vi "Optimiertes Array zusammenstutzen.vi"(6 "Speicher Freigeben":bool, 8 "Zeitstempeln":timestamp[](array[timestamp]), 10 "Anzahl Elemente":i32, 11 "Messdaten":sgl[][](array[numeric])) -> (0 "Zeitstempeln":timestamp[](array[timestamp]), 3 "Messdaten":sgl[][](array[numeric]))   [LabVIEW 2020, in "Messdaten.lvlib"]
uses:
  Messdaten.lvlib
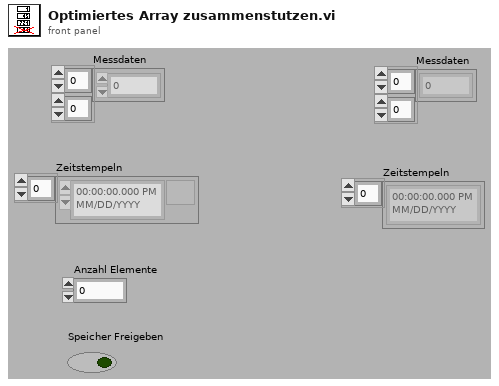
[diagram p1: front panel]
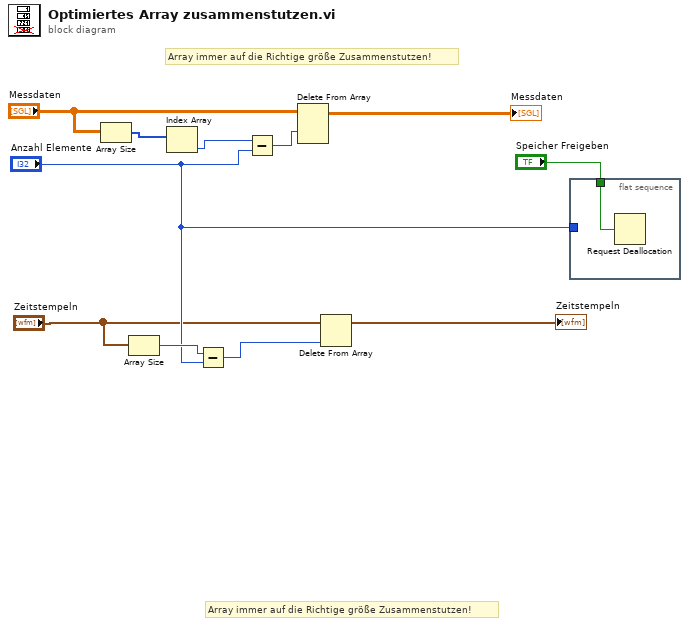
[diagram p0: block diagram]
diagram:
  # "Array immer auf die Richtige größe Zusammenstutzen!"
  # "Array immer auf die Richtige größe Zusammenstutzen!"
  n1 = Array Size(array="Messdaten") -> (size(s)=w8:i32[])
  n2 = Array Size(array="Zeitstempeln") -> (size(s)=w4:i32)
  n3 = Index Array(array=w8) -> (element=w7:i32)  [unwired: 1 in]
  n4 = Subtract(x=w4, y="Anzahl Elemente") -> (x-y=w1:i32)
  n5 = Subtract(x=w7, y="Anzahl Elemente") -> (x-y=w5:i32)
  n6 = Delete From Array(array="Messdaten", index (row)=w5) -> (array with subset deleted=→"Messdaten":sgl[][])  [unwired: 2 in, 1 out]
  n7 = Delete From Array(array="Zeitstempeln", index=w1) -> (array with subset deleted=→"Zeitstempeln":timestamp[])  [unwired: 1 in, 1 out]
  n8 = flat-sequence {
    tunnel: "Anzahl Elemente" -> [_]
    tunnel: "Speicher Freigeben" -> [w12]
    frame #0 {
      n9 = Request Deallocation(w12) -> ()
    }
  }
